vi "Initialise.vi"(8 "error in (no error)":errorcluster, 10 "Data Folder":path, 11 "Data Manager in":refnum<class "Data Manager.lvclass">) -> (0 "error out":errorcluster, 1 "History":T1={"Record Headers"=["Athlete", "Team", "Type", "Date", "Distance", "Moving Time", "Elapsed Time", "Total Elevation Gain"], "All Records"=[]}, 2 "Athlete Profile Map":map{T2, T3}(c390), 3 "Data Manager out":refnum<class "Data Manager.lvclass">)   [LabVIEW 2020, in "Data Manager.lvclass"]
uses:
  Data Manager.lvclass
  Name--cluster.ctl
  Profile--cluster.ctl
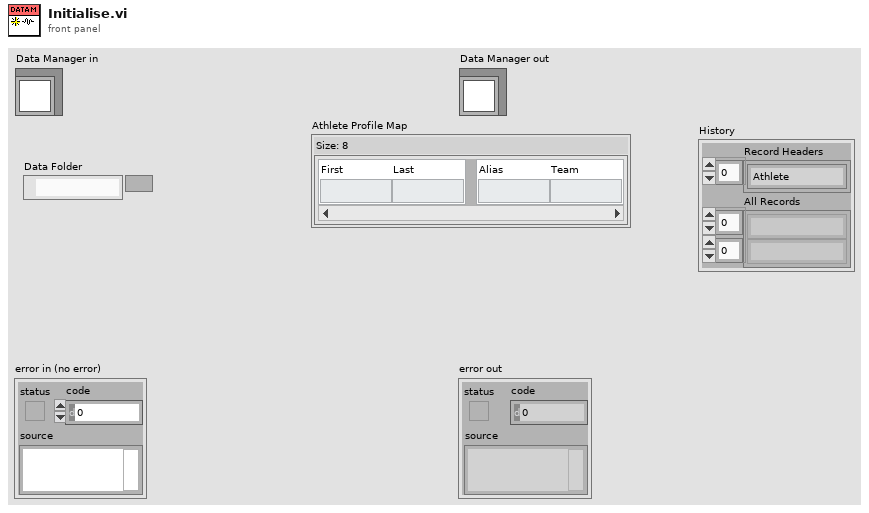
[diagram p1: front panel]
types:
  T1 = cluster{"Record Headers":string[], "All Records":string[][]}
  T2 = typedef "Data Manager.lvclass/Name--cluster.ctl" = cluster{"First":string, "Last":string}
  T3 = typedef "Data Manager.lvclass/Profile--cluster.ctl" = cluster{"Alias":string, "Team":string}
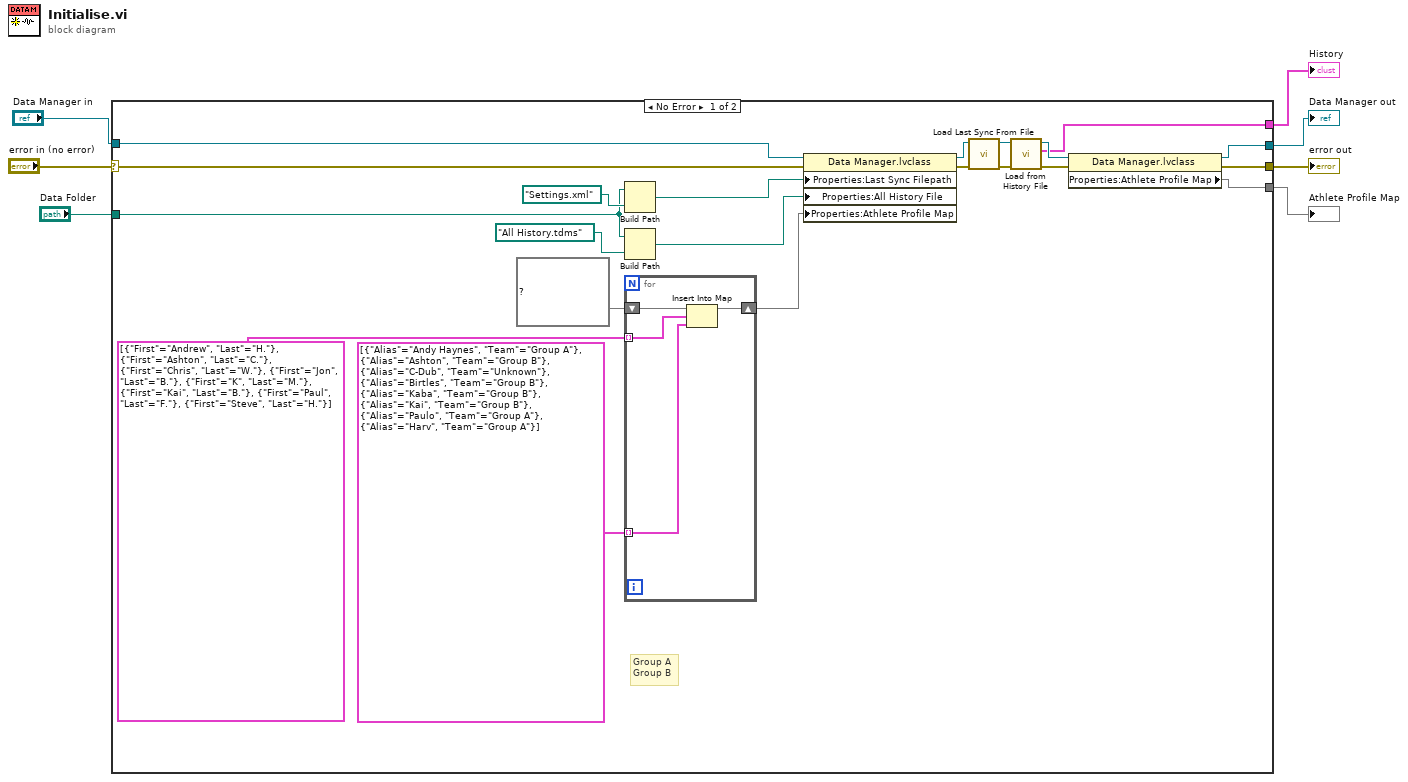
[diagram p0: block diagram]
diagram:
  n1 = case shown="No Error" "error in (no error)" {
    selector: "error in (no error)" -> [w18 w34]
    tunnel: [w15 w34] -> w6
    tunnel: [w14 w33] -> w4
    tunnel: "Data Manager in" -> [w26 w33]
    tunnel: "Data Folder" -> [w22 _]
    tunnel: [w9 _] -> w2
    tunnel: [w8 _] -> w1
    frame No Error {
      # "Group A\nGroup B"
      n2 = Build Path(base path=w22, name or relative path=path "Settings.xml") -> (appended path=w24:path)
      n3 = Build Path(base path=w22, name or relative path=path "All History.tdms") -> (appended path=w23:path)
      n4 = for {
        tunnel: T2[] [{"First"="Andrew", "Last"="H."}, {"First"="Ashton", "Last"="C."}, {"First"="Chris", "Last"="W."}, {"First"="Jon", "Last"="B."}, {"First"="K", "Last"="M."}, {"First"="Kai", "Last"="B."}, {"First"="Paul", "Last"="F."}, {"First"="Steve", "Last"="H."}] ("Names") -> [w30] mode=indexing
        shift-right: [w31] -> w10
        shift-left: map{T2, T3} {} ("Athlete Profile Map") -> [w32]
        tunnel: T3[] [{"Alias"="Andy Haynes", "Team"="Group A"}, {"Alias"="Ashton", "Team"="Group B"}, {"Alias"="C-Dub", "Team"="Unknown"}, {"Alias"="Birtles", "Team"="Group B"}, {"Alias"="Kaba", "Team"="Group B"}, {"Alias"="Kai", "Team"="Group B"}, {"Alias"="Paulo", "Team"="Group A"}, {"Alias"="Harv", "Team"="Group A"}] ("Profile") -> [w29] mode=indexing
        n5 = Insert Into Map(map in=w32, key=w30, value=w29) -> (map out=w31:map{T2, T3})  [unwired: 2 out]
      }
      n6 = property class="Data Manager.lvclass"(reference=w26, error in=w18, "Properties:Last Sync Filepath"=w24, "Properties:All History File"=w23, "Properties:Athlete Profile Map"=w10) -> (reference out=w25:refnum<class "Data Manager.lvclass">, error out=w21:errorcluster)
      n7 = call-dynamic "Load Last Sync From File.vi"("error in (no error)"=w21, "Data Manager in"=w25) -> ("error out"=w19:errorcluster, "Data Manager out"=w20:refnum<class "Data Manager.lvclass">)  [unwired: 8 in]
      n8 = call-dynamic "Load from History File.vi"("error in (no error)"=w19, "Data Manager in"=w20) -> ("error out"=w16:errorcluster, "History"=w8:T1, "Data Manager out"=w17:refnum<class "Data Manager.lvclass">)  [unwired: 7 in]
      n9 = property class="Data Manager.lvclass"(reference=w17, error in=w16) -> (reference out=w14:refnum<class "Data Manager.lvclass">, error out=w15:errorcluster, "Properties:Athlete Profile Map"=w9:map{T2, T3})
    }
    frame Error {
    }
  }
  "error out" <- w6
  "Data Manager out" <- w4
  "Athlete Profile Map" <- w2
  "History" <- w1
